vi "FoodInfo.vi"() -> (0 "食品信息":cluster{"ID":dbl, "食品名称":string, "价格":dbl})   [LabVIEW 2013, in "FoodBase.lvclass"]
doc: "该模板用于创建子VI。"
uses:
  FoodBase.lvclass
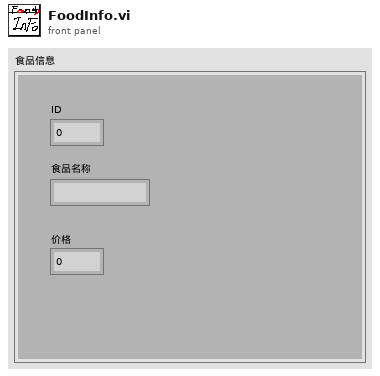
[diagram p1: front panel]
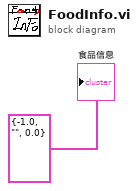
[diagram p0: block diagram]
diagram:
  "食品信息" <- cluster{"ID":dbl, "食品名称":string, "价格":dbl} {"ID"=-1.0, "食品名称"="", "价格"=0.0} ("食品信息 2")
